vi "HEWH Determine Totalized Flow.vi"(0 "Highest Volume Index":i32, 1 "Sub Array End Index":i32, 5 "Draw Start":i32, 11 "error in (no error)":errorcluster) -> (4 "Zero Start Index":i32, 6 "Zero End Index":i32, 10 "End Index":i32, 15 "error out":errorcluster)   [LabVIEW 2023]
panel:
  # "This is the index of the maxium value"
  # "Zero the data at these and between\nthese indexes"
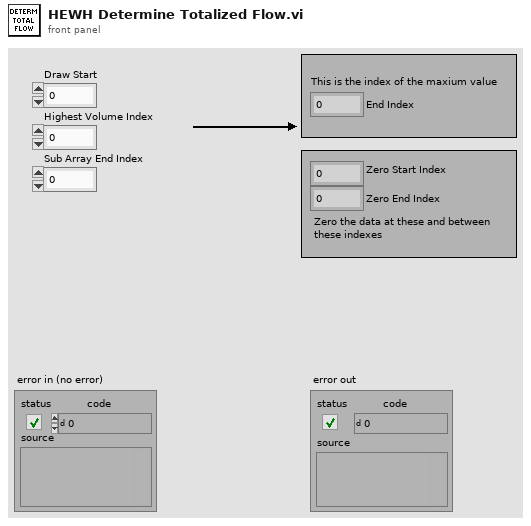
[diagram p1: front panel]
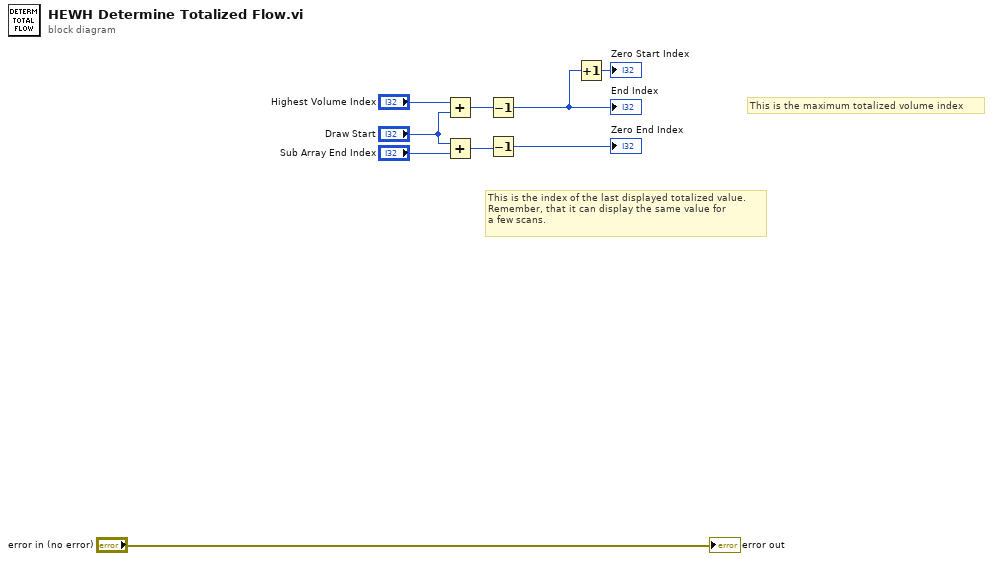
[diagram p0: block diagram]
diagram:
  # "This is the index of the last displayed totalized value. \nRemember, that it can display the same value for\na few scans."
  # "This is the maximum totalized volume index"
  n1 = Add(x="Highest Volume Index", y="Draw Start") -> (x+y=w4:i32)
  n2 = Add(x="Draw Start", y="Sub Array End Index") -> (x+y=w8:i32)
  n3 = Decrement(x=w4) -> (x-1=w2:i32)
  "End Index" <- w2
  n4 = Decrement(x=w8) -> (x-1=→"Zero End Index":i32)
  n5 = Increment(x=w2) -> (x+1=→"Zero Start Index":i32)
  "error out" <- "error in (no error)"
